vi "Square Waveform.vi"(4 "duty cycle (%)":dbl=50.0 format="%0.2f", 5 "offset":dbl format="%0.2p", 6 "sampling info":cluster{"Fs":dbl, "#s":dbl}={"Fs"=1000.0, "#s"=1000.0} {"Fs" format="%.2p"}, 7 "reset signal":bool, 8 "error in (no error)":errorcluster, 9 "phase":dbl format="%.2p", 10 "amplitude":dbl=1.0 format="%0.2p", 11 "frequency":dbl=10.0 format="%0.2p") -> (0 "error out":errorcluster, 3 "signal out":waveform(dbl))   [LabVIEW 2020, in "NI_MABase.lvlib"]
doc: "Generates a waveform containing a square wave."
uses:
  NI_MABase.lvlib
  NI_AALBase.lvlib
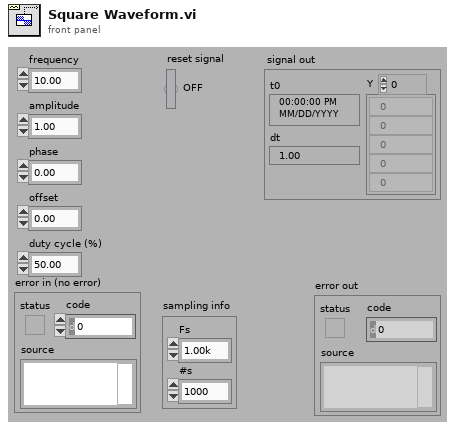
[diagram p1: front panel]
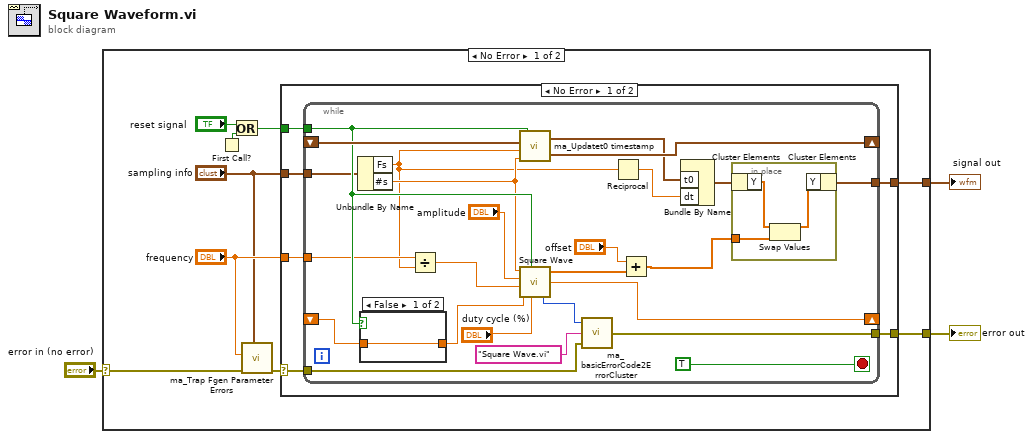
[diagram p0: block diagram]
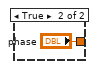
[diagram p2: hidden frame]
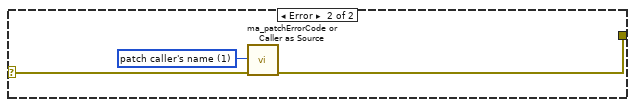
[diagram p3: hidden frame]
diagram:
  n1 = case shown="No Error" "error in (no error)" {
    selector: "error in (no error)" -> [w5 w52]
    tunnel: [w8 w52] -> w3
    tunnel: [w4 _] -> w1
    frame No Error {
      n2 = First Call?() -> (First Call?: T/F=w6:bool)
      n3 = Or(x="reset signal", y=w6) -> (x .or. y?=w11:bool)
      n4 = call "ma_Trap Fgen Parameter Errors.vi"("Sampling info"="sampling info", "error in (no error)"=w5, "frequency"="frequency") -> ("error out"=w10:errorcluster)  [unwired: 8 in]
      n5 = case shown="No Error" w10 {
        selector: w10 -> [w14 w51]
        tunnel: w11 -> [w18 _]
        tunnel: "sampling info" -> [w17 _]
        tunnel: "frequency" -> [w16 _]
        tunnel: [w15 w50] -> w8
        tunnel: [w13 _] -> w4
        frame No Error {
          n6 = while {
            tunnel: w14 -> [w24]
            tunnel: [w26] -> w15
            tunnel: w16 -> [w27]
            tunnel: w17 -> [w28]
            tunnel: w18 -> [w31]
            shift-left: _ -> [w34]
            shift-right: [w36] -> _
            shift-left: _ -> [w40]
            shift-right: [w39] -> _
            tunnel: [w20] -> w13
            stop <- TRUE stop-if-true
            n7 = Unbundle By Name(w28) -> ("Fs"=w19:dbl, "#s"=w29:dbl)
            n8 = case shown="False" w31 {
              tunnel: [w47 "phase"] -> w35
              tunnel: w34 -> [w47 _]
              frame False {
              }
              frame True {
              }
            }
            n9 = Divide(x=w27, y=w19) -> (x/y=w30:dbl)
            n10 = call "ma_Updatet0 timestamp.vi"("samples"=w29, "sampling rate (S/s)"=w19, "tf previous"=w40, "Reset Generation"=w31) -> ("tf new"=w39:timestamp, "t0"=w23:timestamp)
            n11 = call "Square Wave.vi"("samples"=w29, "reset phase"=w31, "amplitude"="amplitude", "frequency"=w30, "duty cycle (%)"="duty cycle (%)", "phase in"=w35) -> ("square wave"=w37:dbl[], "phase out"=w36:dbl, "error"=w43:i32)
            n12 = call "ma_basicErrorCode2ErrorCluster.vi"("error in (no error)"=w24, "subVI name"="Square Wave.vi" ("subVI Name"), "Error Code"=w43) -> ("error out"=w26:errorcluster)
            n13 = Reciprocal(x=w19) -> (1/x=w33:dbl)
            n14 = Add(x="offset", y=w37) -> (x+y=w21:dbl[])
            n15 = Bundle By Name("t0"=w23, "dt"=w33) -> (w22:waveform(dbl))  [unwired: 1 in]
            n16 = in-place {
              in-place-border: w21 -> [w44]
              n17 = in-place-cluster #1(w22) -> ("Y"=w46:dbl[])
              n18 = Swap Values(12:w46, 14:w44) -> (1:w45:dbl[])  [unwired: 1 in, 1 out]
              n19 = in-place-cluster #1("Y"=w45) -> (w20:waveform(dbl))
            }
          }
        }
        frame Error {
          w49 = u16 1 items=["patch error code", "patch caller's name"] ("operation")
          n20 = call "ma_patchErrorCode or Caller as Source.vi"("error in (no error)"=w51, "operation"=w49) -> ("error out"=w50:errorcluster)  [unwired: 9 in]
        }
      }
    }
    frame Error {
    }
  }
  "error out" <- w3
  "signal out" <- w1
